vi "Get RTPath String.vi"(7 "SysDef Log File Path":path, 8 "error in (no error)":errorcluster, 11 "Target OS in":string) -> (0 "error out":errorcluster, 1 "RT Folder Path":string, 2 "RT File Path":string, 3 "Target OS out":string)   [LabVIEW 2026, in "Telemetry System Tests.lvclass"]
uses:
  Telemetry System Tests.lvclass
  Telemetry Test Utilities/Telemetry Test Utilities.lvlib
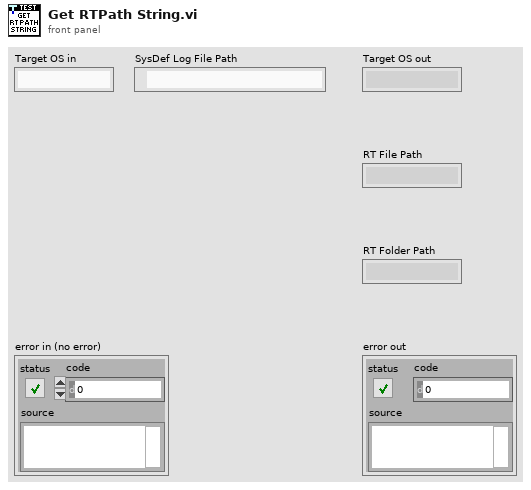
[diagram p1: front panel]
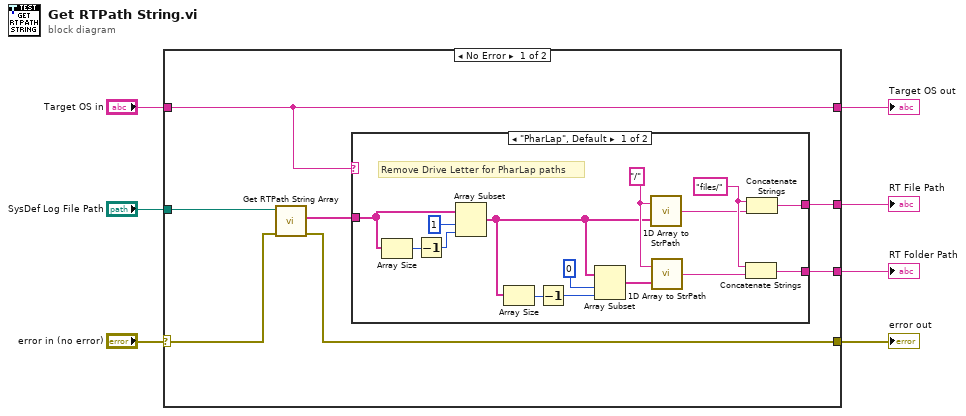
[diagram p0: block diagram]
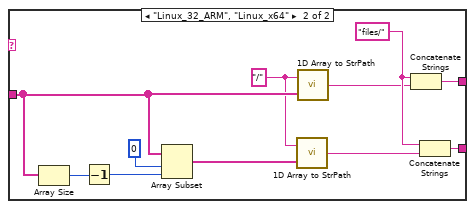
[diagram p2: hidden frame]
diagram:
  n1 = case shown="No Error" "error in (no error)" {
    selector: "error in (no error)" -> [w11 w41]
    tunnel: [w14 _] -> w7
    tunnel: [w13 w41] -> w6
    tunnel: "Target OS in" -> [w8 w42]
    tunnel: [w8 w42] -> w3
    tunnel: [w10 _] -> w2
    tunnel: "SysDef Log File Path" -> [w9 _]
    frame No Error {
      n2 = call "Get RTPath String Array.vi"("error in (no error)"=w11, "SysDef Log File Path"=w9) -> ("error out"=w13:errorcluster, "File Path String Array"=w12:string[])  [unwired: 8 in]
      n3 = case shown="\"PharLap\", Default" w8 {
        tunnel: w12 -> [w22 w36]
        tunnel: [w29 w40] -> w14
        tunnel: [w24 w37] -> w10
        frame "PharLap", Default {
          w25 = "files/" ("string")
          w27 = "/" ("delimiter (Tab)")
          # "Remove Drive Letter for PharLap paths"
          n4 = Array Size(array=w22) -> (size(s)=w21:i32)
          n5 = Decrement(x=w21) -> (x-1=w20:i32)
          n6 = Array Subset(array=w22, index=1, length=w20) -> (w15:string[])
          n7 = Array Size(array=w15) -> (size(s)=w18:i32)
          n8 = Decrement(x=w18) -> (x-1=w19:i32)
          n9 = Array Subset(array=w15, index=0, length=w19) -> (w16:string[])
          n10 = call "1D Array to StrPath.vi"("File Path String Array"=w15, "Delimiter"=w27) -> ("Path string"=w23:string)
          n11 = call "1D Array to StrPath.vi"("File Path String Array"=w16, "Delimiter"=w27) -> ("Path string"=w26:string)
          n12 = Concatenate Strings(w25, w26) -> (w24:string)
          n13 = Concatenate Strings(w25, w23) -> (w29:string)
        }
        frame "Linux_32_ARM", "Linux_x64" {
          w34 = "/" ("Delimiter")
          w38 = "files/" ("string")
          n14 = Array Size(array=w36) -> (size(s)=w31:i32)
          n15 = Decrement(x=w31) -> (x-1=w30:i32)
          n16 = Array Subset(array=w36, index=0, length=w30) -> (w35:string[])
          n17 = call "1D Array to StrPath.vi"("File Path String Array"=w35, "Delimiter"=w34) -> ("Path string"=w32:string)
          n18 = call "1D Array to StrPath.vi"("File Path String Array"=w36, "Delimiter"=w34) -> ("Path string"=w33:string)
          n19 = Concatenate Strings(w38, w33) -> (w40:string)
          n20 = Concatenate Strings(w38, w32) -> (w37:string)
        }
      }
    }
    frame Error {
    }
  }
  "RT File Path" <- w7
  "error out" <- w6
  "Target OS out" <- w3
  "RT Folder Path" <- w2
